vi "External Sensor Display Names DAO.vi"(7 "refnum":T1, 8 "error in (no error)":errorcluster, 10 "Display Name In":string[](array[string]), 11 "Persistent DAO Actions":T2) -> (0 "error out":errorcluster, 2 "Display Name Out":string[](array[string]), 4 "refnum out":T1)   [LabVIEW 2013]
uses:
  Metadata/Persistant DAO Actions.ctl
  <vilib>/Utility/config.llb/Config Data RefNum.ctl
  <vilib>/Utility/config.llb/NI_LVConfig.lvlib
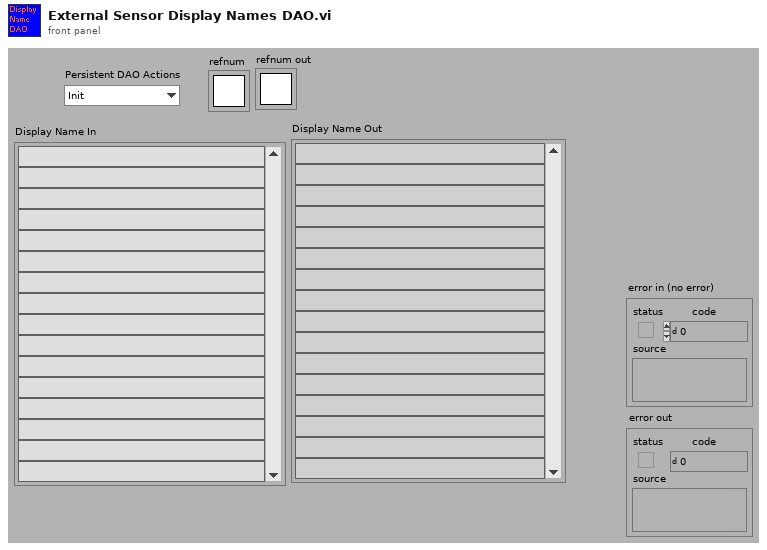
[diagram p1: front panel]
types:
  T1 = typedef "NI_LVConfig.lvlib/Config Data RefNum.ctl" = refnum<k1>
  T2 = typedef "Persistant DAO Actions.ctl" = enum16{"Init", "Get", "Set", "Load", "Save"}
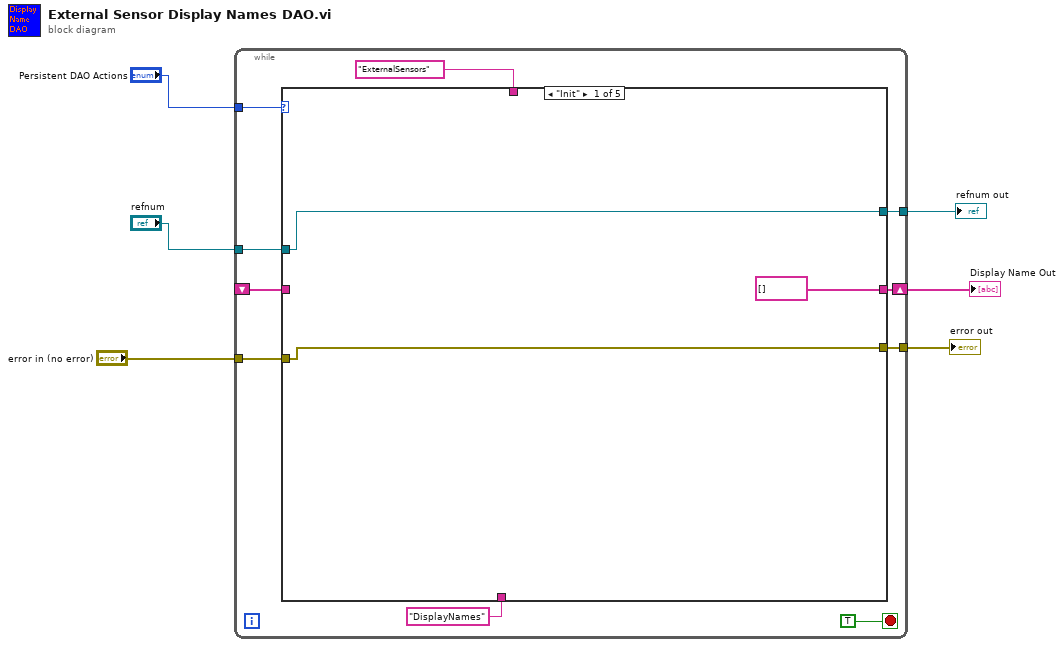
[diagram p0: block diagram]
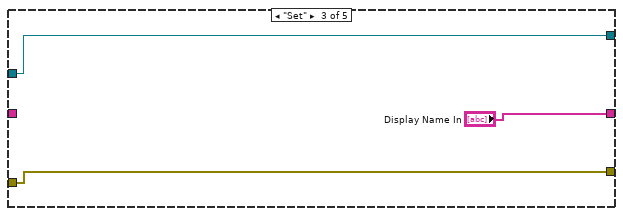
[diagram p3: hidden frame]
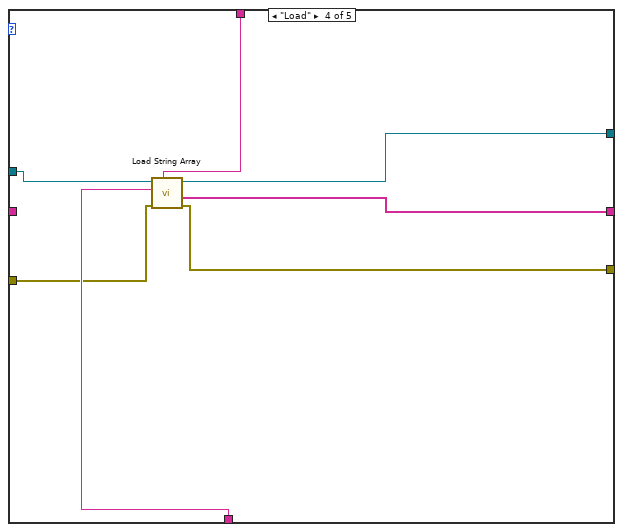
[diagram p4: hidden frame]
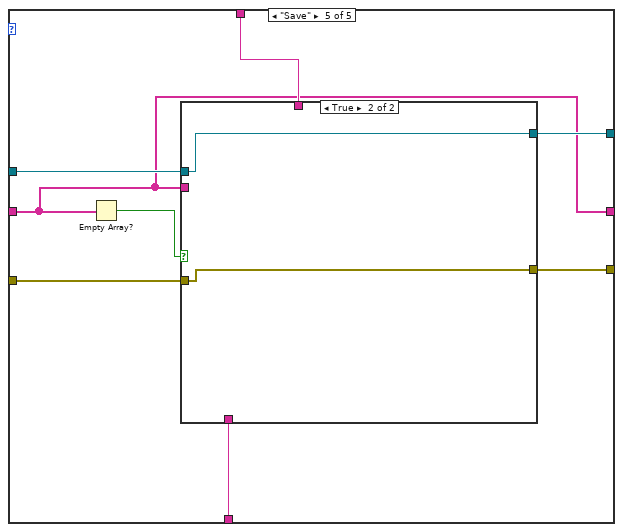
[diagram p5: hidden frame]
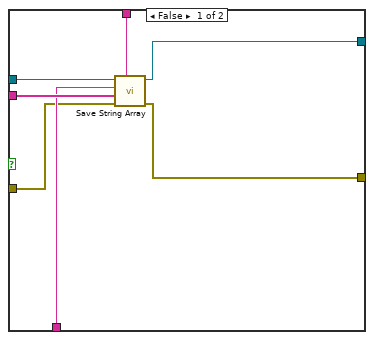
[diagram p6: hidden frame]
diagram:
  n1 = while {
    tunnel: "Persistent DAO Actions" -> [w15]
    shift-right: [w14] -> w5
    shift-left: _ -> [w13]
    tunnel: "refnum" -> [w12]
    tunnel: "error in (no error)" -> [w9]
    tunnel: [w8] -> w2
    tunnel: [w7] -> w1
    stop <- TRUE stop-if-true
    n2 = case shown="\"Init\"" w15 {
      tunnel: [string[] [] ("String Array Out") w22 "Display Name In" w26 w33] -> w14
      tunnel: w13 -> [_ w22 _ _ w33]
      tunnel: w12 -> [w19 w21 w24 w30 w39]
      tunnel: "DisplayNames" -> [_ _ _ w32 w38]
      tunnel: "ExternalSensors" -> [_ _ _ w31 w37]
      tunnel: w9 -> [w18 w20 w23 w28 w36]
      tunnel: [w19 w21 w24 w29 w35] -> w8
      tunnel: [w18 w20 w23 w27 w34] -> w7
      frame "Init" {
      }
      frame "Get" {
      }
      frame "Set" {
      }
      frame "Load" {
        n3 = call "Load String Array.vi"("section"=w31, "error in (no error)"=w28, "key"=w32, "refnum"=w30) -> ("error out"=w27:errorcluster, "String Array Out"=w26:string[], "refnum out"=w29:T1)  [unwired: 5 out]
      }
      frame "Save" {
        n4 = Empty Array?(array=w33) -> (empty?=w40:bool)
        n5 = case shown="True" w40 {
          tunnel: w33 -> [w47 _]
          tunnel: w39 -> [w46 w49]
          tunnel: w38 -> [w45 _]
          tunnel: w37 -> [w44 _]
          tunnel: w36 -> [w43 w48]
          tunnel: [w42 w49] -> w35
          tunnel: [w41 w48] -> w34
          frame False {
            n6 = call "Save String Array.vi"("section"=w44, "error in (no error)"=w43, "String Array In"=w47, "key"=w45, "refnum"=w46) -> ("error out"=w41:errorcluster, "refnum out"=w42:T1)  [unwired: 5 out]
          }
          frame True {
          }
        }
      }
    }
  }
  "Display Name Out" <- w5
  "refnum out" <- w2
  "error out" <- w1
